vi "Reset USB&temp v 1.vi"() -> (0 "Reset Error":bool)   [LabVIEW 2017]
uses:
  <vilib>/Platform/TimedLoop/XDataNode/timing_clust.ctl
  <vilib>/Platform/TimedLoop/XDataNode/nitl_modes.ctl
  <vilib>/Platform/TimedLoop/XDataNode/wakeup.ctl
  <vilib>/platform/TimedLoop/XDataNode/XDataNode.xnode
  <vilib>/Platform/TimedLoop/XDataNode/XDNodeRunTimeDep.lvlib
panel:
  out "Reset Time Out":dbl
  out "Message":string
  in  "End Reset Routine":bool
  # "RESET USB $ TEMP"
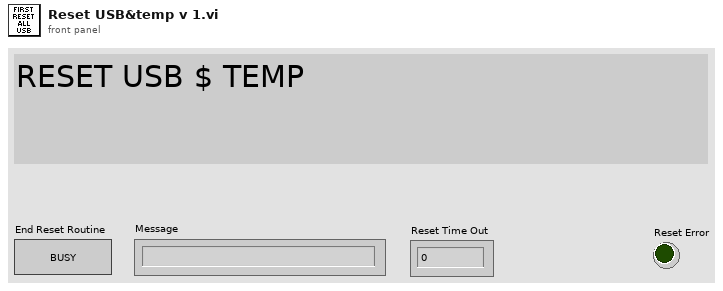
[diagram p1: front panel]
types:
  T1 = typedef "XDNodeRunTimeDep.lvlib/timing_clust.ctl" = cluster{"Expected End [f-1]":u64, "Actual End [f-1]":u64, "Finished Late? [f-1]":bool, "Expected End [i-1]":u64, "Actual End [i-1]":u64, "Finished Late? [i-1]":bool, "Expected Start [i]":u64, "Actual Start [i]":u64, "Expected Start [f]":u64, "Actual Start [f]":u64, "Source Name":string, "Structure Name":string, "Period":i64, "Deadline":i64, "Offset":i64, "Start":i64, "Priority":i32, "Timeout":i32, "Mode":T2, "Wakeup Reason":T3, "Error":errorcluster, "Source Type":string, "Secondary Source Type":string, "Global End Time":u64, "Global Start Time":u64, "Frame Duration":u64, "Iteration Duration":u64, "Assigned CPU":i32, "I/O Scan Engine Mode":u32}
  T2 = typedef "XDNodeRunTimeDep.lvlib/nitl_modes.ctl" = enum32{"No Change", "Process missed periods, maintain original phase", "Discard missed periods, maintain original phase", "Process missed periods, ignore original phase", "Discard missed periods, ignore original phase"}
  T3 = typedef "XDNodeRunTimeDep.lvlib/wakeup.ctl" = enum32{"Normal", "Aborted", "Asynchronous wakeup", "Timing source error", "Timed loop error", "Timeout"}
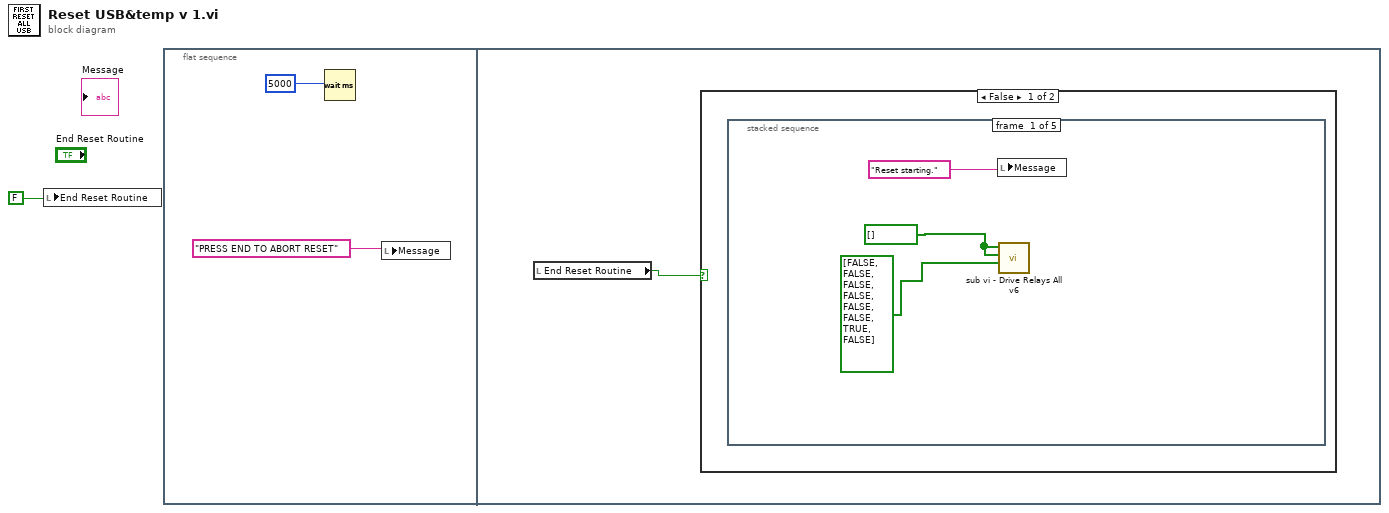
[diagram p0: block diagram]
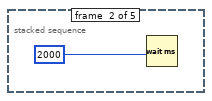
[diagram p2: hidden frame]
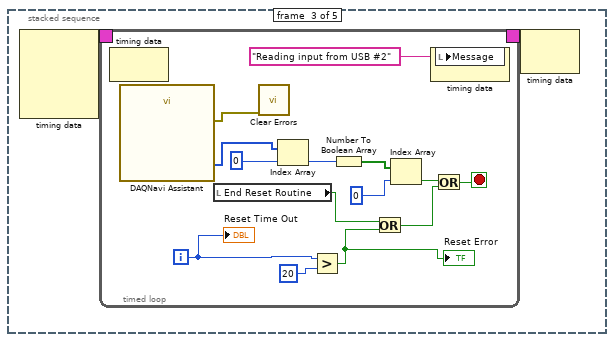
[diagram p3: hidden frame]
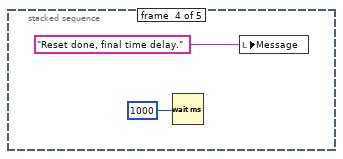
[diagram p4: hidden frame]
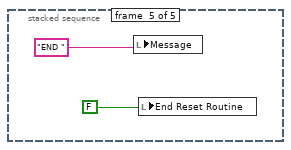
[diagram p5: hidden frame]
diagram:
  n1 = local write "End Reset Routine"(FALSE) -> ()
  n2 = flat-sequence {
    frame #0 {
      n3 = Wait (ms)(milliseconds to wait=5000) -> ()  [unwired: 1 out]
      n4 = local write "Message"("PRESS END TO ABORT RESET") -> ()
    }
    frame #1 {
      n5 = local read "End Reset Routine"() -> (w4:bool)
      n6 = case shown="False" w4 {
        frame False {
          n7 = stacked-sequence {
            frame #0 {
              w6 = bool[] []
              n8 = local write "Message"("Reset starting.") -> ()
              n9 = call "sub vi - Drive Relays All v6.vi"("Array #2"=bool[] [FALSE, FALSE, FALSE, FALSE, FALSE, FALSE, TRUE, FALSE], "Array #1"=w6, "Array #0"=w6) -> ()  [unwired: 8 in, 1 out]
            }
            frame #1 {
              n10 = Wait (ms)(milliseconds to wait=2000) -> ()  [unwired: 1 out]
            }
            frame #2 {
              n11 = node-c288() -> (w10:T1)  [unwired: 4 in]
              n12 = timed-loop {
                timing: w10 -> [_]
                timing-out: [_] -> w9
                i -> [w11]
                stop <- w20 stop-if-true
                n13 = node-c288() -> ()  [unwired: 1 in, 1 out]
                n14 = call "DAQNavi Assistant"() -> ("error out"=w16:errorcluster, "dataOut(U8Array)"=w17:u8[])  [unwired: 26 in]
                n15 = local read "End Reset Routine"() -> (w15:bool)
                n16 = call <vilib>:"Clear Errors.vi"("error in (no error)"=w16) -> ()  [unwired: 5 in, 2 out]
                n17 = Index Array(array=w17, index=0) -> (element=w22:u8)
                n18 = Greater?(x=w11, y=20) -> (0:w12:bool)
                "Reset Error" <- w12
                n19 = Number To Boolean Array(number=w22) -> (Boolean array=w23:bool[])
                n20 = Or(x=w15, y=w12) -> (x .or. y?=w13:bool)
                n21 = Index Array(array=w23, index=0) -> (element=w19:bool)
                n22 = node-c288() -> ()  [unwired: 1 in, 1 out]
                n23 = Or(x=w19, y=w13) -> (x .or. y?=w20:bool)
                n24 = local write "Message"("Reading input from USB #2") -> ()
                "Reset Time Out" <- w11
              }
              n25 = node-c288(w9) -> ()  [unwired: 1 out]
            }
            frame #3 {
              n26 = Wait (ms)(milliseconds to wait=1000) -> ()  [unwired: 1 out]
              n27 = local write "Message"("Reset done, final time delay.") -> ()
            }
            frame #4 {
              n28 = local write "Message"("END ") -> ()
              n29 = local write "End Reset Routine"(FALSE) -> ()
            }
          }
        }
        frame True {
        }
      }
    }
  }
